vi "Initialization Test.vi"() -> ()   [LabVIEW 2015, in "Wait On Boolean Step.lvclass"]
uses:
  Runtime/Wait On Boolean Step.lvclass
  <vilib>/NI/Tag Bus Module Framework/channel/TBM channel.lvclass
  classes/Step/Config/Step Config.lvclass
  <vilib>/NI/Tag Bus/tag/Data Type.ctl
  <vilib>/NI/Tag Bus Module Framework/channel/channel classification.ctl
  Config/Wait On Boolean Step Config.lvclass
  module/configuration/Sequencer Module configuration.lvclass
  module/configuration/Line.ctl
  classes/Sequence/Config/Sequence Config.lvclass
  module/execution/Sequencer Module runtime.lvclass
  Config/Wait On Boolean Step Config.lvclass/Wait On Boolean Step Config.ctl
  <vilib>/NI/Tag Bus/tag/tag descriptor.lvclass/tag descriptor.ctl
  Config/Write Wait On Boolean Event.vi
  classes/Sequence/Config/Read Size.vi
  <vilib>/NI/Tag Bus/tag/tag descriptor.lvclass
  <vilib>/NI/Configuration Framework/serializable configuration/NISE_CEF_serializable configuration.lvclass
panel:
  out "Size":i32
  out "Steps":refnum<class "Step Config.lvclass">[](array[class])
  out "Name 2":string
  out "error out":errorcluster
  out "Channels":refnum<class "TBM channel.lvclass">[](array[class])
  out "Channel Names":string[](array[string])
  in  "Name":string="Led Sequence"
  in  "Jump Tag Name":string="Boolean processing result 0"
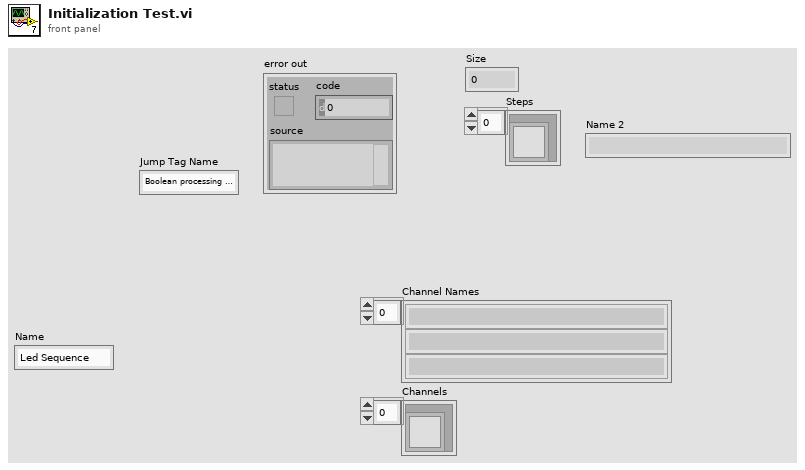
[diagram p1: front panel]
types:
  T1 = typedef "Sequencer Module configuration.lvclass/Line.ctl" = cluster{"Sequence":refnum<class "Sequence Config.lvclass">}
  T2 = typedef "TBM channel.lvclass/channel classification.ctl" = enum16{"input data", "output data", "processing parameter", "processing result"}
  T3 = typedef "tag bus.lvlib/tag descriptor.lvclass/Data Type.ctl" = enum16{"Double", "Single", "I64", "I32", "I16", "I8", "U64", "U32", "U16", "U8", "Boolean", "String", "Array of Double", "Array of Single", "Array of I64", "Array of I32", "Array of I16", "Array of I8", "Array of U64", "Array of U32", "Array of U16", "Array of U8", "Array of Boolean", "Array of String"}
  T4 = typedef "TBM channel.lvclass/data tables.ctl" = cluster{"input data":T5, "processing parameter":T5, "processing result":T5, "output data":T5}
  T5 = typedef "tag bus.lvlib/dictionary table pair.ctl" = cluster{"data dictionary":refnum<class "data dictionary.lvclass">, "data table":T6}
  T6 = typedef "tag bus.lvlib/data table.lvlib/data table.ctl" = cluster{"Double":dbl[], "Single":sgl[], "I64":i64[], "I32":i32[], "I16":i16[], "I8":i8[], "U64":u64[], "U32":u32[], "U16":u16[], "U8":u8[], "Boolean":bool[], "String":string[], "Array of Double":cluster{"DBL Array":dbl[]}[], "Array of Single":cluster{"SGL Array":sgl[]}[], "Array of I64":cluster{"I64 Array":i64[]}[], "Array of I32":cluster{"I32 Array":i32[]}[], "Array of I16":cluster{"I16 Array":i16[]}[], "Array of I8":cluster{"I8 Array":i8[]}[], "Array of U64":cluster{"U64 Array":u64[]}[], "Array of U32":cluster{"U32 Array":u32[]}[], "Array of U16":cluster{"U16 Array":u16[]}[], "Array of U8":cluster{"U8 Array":u8[]}[], "Array of Boolean":cluster{"Boolean Array":bool[]}[], "Array of String":cluster{"String Array":string[]}[]}
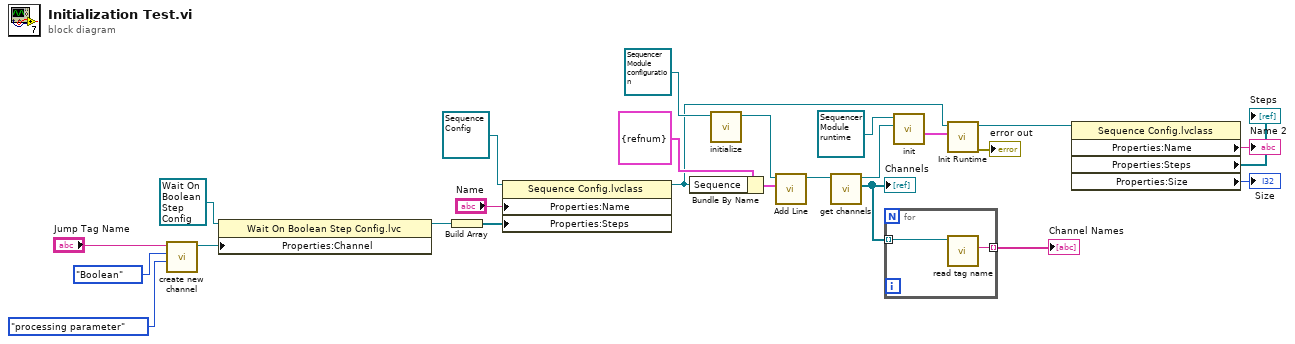
[diagram p0: block diagram]
diagram:
  n1 = call <vilib>:"create new channel.vi"("channel classification"=channel_classification."processing parameter", "data type"=Data_Type."Boolean" ("Data Type"), "channel name"="Jump Tag Name") -> ("channel"=w22:refnum<class "TBM channel.lvclass">)  [unwired: 8 in]
  n2 = property class="Wait On Boolean Step Config.lvc"(reference=refnum<class "Wait On Boolean Step Config.lvclass"> refnum ("Wait On Boolean Step Config.lvclass"), "Properties:Channel"=w22) -> (reference out=w14:refnum<class "Wait On Boolean Step Config.lvclass">)  [unwired: 1 in, 1 out]
  n3 = Build Array(w14) -> (w15:refnum<class "Wait On Boolean Step Config.lvclass">[])
  n4 = property class="Sequence Config.lvclass"(reference=refnum<class "Sequence Config.lvclass"> refnum ("Sequence Config.lvclass"), "Properties:Name"="Name", "Properties:Steps"=w15) -> (reference out=w9:refnum<class "Sequence Config.lvclass">)  [unwired: 1 in, 1 out]
  n5 = Bundle By Name(cluster=T1 {"Sequence"=refnum} ("Line"), "Sequence"=w9) -> (w17:T1)
  n6 = call <vilib>:"initialize.vi"("configuration in"=refnum<class "Sequencer Module configuration.lvclass"> refnum ("tag bus configurable plugin module configuration")) -> ("configuration out"=w19:refnum<class "Sequencer Module configuration.lvclass">)  [unwired: 8 in, 2 out]
  n7 = call "Add Line.vi"("Line"=w17, "Sequencer Module configuration in"=w19) -> ("Sequencer Module configuration out"=w12:refnum<class "Sequencer Module configuration.lvclass">)  [unwired: 7 in, 2 out]
  n8 = call-dynamic "get channels.vi"("Sequencer Module configuration in"=w12) -> ("channels"=w11:refnum<class "TBM channel.lvclass">[], "Sequencer Module configuration out"=w7:refnum<class "Sequencer Module configuration.lvclass">)  [unwired: 9 in]
  "Channels" <- w11
  n9 = for {
    tunnel: w11 -> [w27] mode=indexing
    tunnel: [w26] -> w10 mode=indexing
    n10 = call <vilib>:"read tag name.vi"("system tag in"=w27) -> ("name"=w26:string)  [unwired: 8 in, 2 out]
  }
  "Channel Names" <- w10
  n11 = call-dynamic "init.vi"("TBM module configuration in"=w7, "Sequencer Module runtime in"=refnum<class "Sequencer Module runtime.lvclass"> refnum ("tag bus configurable plugin module")) -> ("data allocations"=w6:T4)  [unwired: 6 in, 3 out]
  n12 = call-dynamic "Init Runtime.vi"("data allocations"=w6, "Sequence Config in"=w9) -> ("error out"=→"error out":errorcluster, "Sequence Config out"=w4:refnum<class "Sequence Config.lvclass">)  [unwired: 7 in, 1 out]
  n13 = property class="Sequence Config.lvclass"(reference=w4) -> ("Properties:Name"=→"Name 2":string, "Properties:Steps"=→"Steps":refnum<class "Step Config.lvclass">[], "Properties:Size"=→"Size":i32)  [unwired: 1 in, 2 out]
